vi "io.command-builder.DO.vi"(8 "error in":errorcluster, 9 "parsed dout state":cluster{"state":bool, "timeoutSeconds":u16}, 10 "IoConf in":T1={"ADDR"=0, "Label"="", "Type"=enum."DI", "Mode"=enum."RIO", "Value"="", "Tags"="", "calibration"=[]} {"calibration"."Y" format="%#.3f"; "calibration"."X" format="%#.3f"; "ADDR" format="%04d"}) -> (0 "error out":errorcluster, 2 "Frameless Command":string)   [LabVIEW 2024]
uses:
  controls/IONode.ctl
  controls/type.address.ctl
  controls/enum.io.type.ctl
  controls/enum.io.mode.ctl
  controls/typeXyPoint.ctl
  controls/enum.io-rio.ctl
  variantCtrlNumber.vi
panel:
  in  "Value in":cluster{"value":u8, "timeoutSeconds":u16}
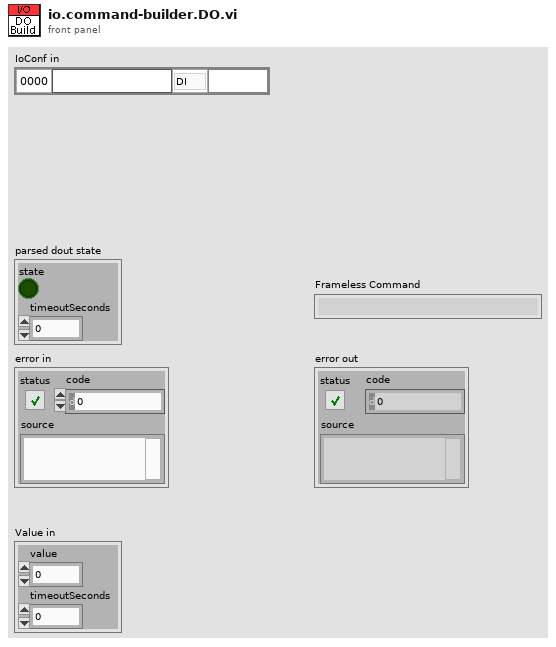
[diagram p1: front panel]
types:
  T1 = typedef "IONode.ctl" = cluster{"ADDR":T2, "Label":string, "Type":T3, "Mode":T4, "Value":string, "Tags":string, "calibration":T5[]}
  T2 = typedef "type.address.ctl" = u16
  T3 = typedef "enum.io.type.ctl" = enum16{"Type", "DI", "DO", "AI", "AO", "VL", "BUF"}
  T4 = typedef "enum.io.mode.ctl" = enum16{"Mode", "RIO", "SIM"}
  T5 = typedef "typeXyPoint.ctl" = cluster{"X":dbl, "Y":dbl}
  T6 = cluster{"DataSize":u8, "Address":u8, "Command(SET-DOUT)":u8, "Channel":u8, "DigVal":bool, "Timeout":u16}
  T7 = typedef "enum.io-rio.ctl" = enum16{"RIO_CALIBRATION"}
  T8 = cluster{"WRITE_DO":u8, "Address":T2, "Channel":u8, "value":u8, "timeoutSeconds":u16}
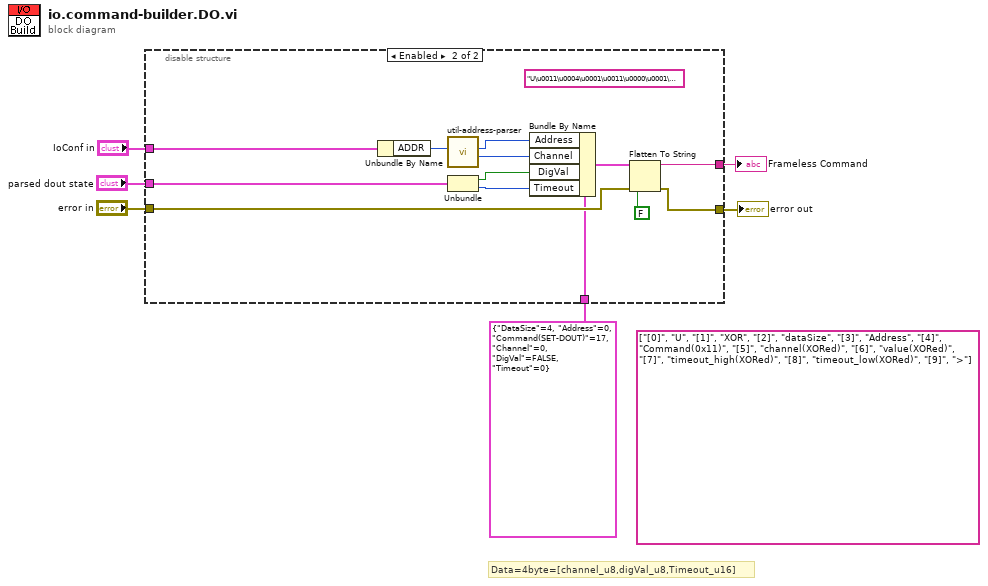
[diagram p0: block diagram]
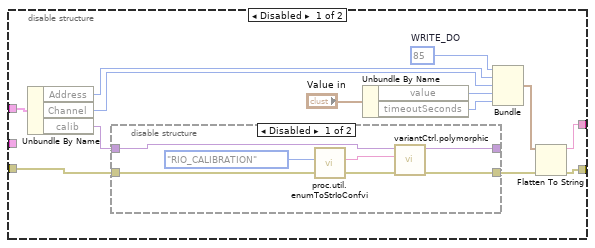
[diagram p2: hidden frame]
diagram:
  (unwired) string[][] [["[0]", "U"], ["[1]", "XOR"], ["[2]", "dataSize"], ["[3]", "Address"], ["[4]", "Command(0x11)"], ["[5]", "channel(XORed)"], ["[6]", "value(XORed)"], ["[7]", "timeout_high(XORed)"], ["[8]", "timeout_low(XORed)"], ["[9]", ">"]] ("Command To RIO")
  # "Data=4byte=[channel_u8,digVal_u8,Timeout_u16]"
  n1 = disable-structure shown="Enabled" {
    disable-tunnel: [w19 w40] -> w6
    disable-tunnel: "IoConf in" -> [w14 w39]
    disable-tunnel: "error in" -> [w12 w38]
    disable-tunnel: [w7 w37] -> w3
    disable-tunnel: "parsed dout state" -> [_ w31]
    disable-tunnel: T6 {"DataSize"=4, "Address"=0, "Command(SET-DOUT)"=17, "Channel"=0, "DigVal"=FALSE, "Timeout"=0} ("cluster") -> [_ w36]
    frame Disabled {
      w11 = u8 85  # WRITE_DO
      n2 = Unbundle By Name(w14) -> ("Address"=w17:T2, "Channel"=w18:u8, "calib"=w16:variant)
      n3 = disable-structure shown="Disabled" {
        disable-tunnel: w16 -> [w25 w27]
        disable-tunnel: [w24 w27] -> _
        disable-tunnel: [w23 w26] -> w15
        disable-tunnel: w12 -> [w20 w26]
        frame Disabled {
          n4 = call "proc.util.enumToStrIoConfvi.vi"("Step var"=enum.io-rio."RIO_CALIBRATION") -> ("String"=w22:string)  [unwired: 10 in]
          n5 = call-poly "variantCtrl.polymorphic.vi"("error in"=w20, "name in"=w22, "variant in"=w25) -> ("error out"=w23:errorcluster, "variant out"=w24:variant)  [unwired: 5 in, 2 out]
        }
        frame Enabled {
        }
      }
      n6 = Unbundle By Name("Value in") -> ("value"=w10:u8, "timeoutSeconds"=w9:u16)
      n7 = Bundle("WRITE_DO"=w11, "Address"=w17, "Channel"=w18, "value"=w10, "timeoutSeconds"=w9) -> (w8:T8)  [unwired: 1 in]
      n8 = Flatten To String(anything=w8, error in (no error)=w15) -> (data string=w19:string, error out=w7:errorcluster)  [unwired: 2 in, 1 out]
    }
    frame Enabled {
      (unwired) "U\u0011\u0004\u0001\u0011\u0000\u0001\u0000\u0000>" ("Command To RIO")
      n9 = Unbundle By Name(w39) -> ("ADDR"=w30:T2)
      n10 = call "util-address-parser.vi"("ADDR 2"=w30) -> ("Channel"=w29:u8, "Address"=w28:u8)  [unwired: 9 in]
      n11 = Unbundle(w31) -> ("state"=w34:bool, "timeoutSeconds"=w35:u16)
      n12 = Bundle By Name(cluster=w36, "Address"=w28, "Channel"=w29, "DigVal"=w34, "Timeout"=w35) -> (w33:T6)
      n13 = Flatten To String(anything=w33, prepend array or string size? (T)=FALSE, error in (no error)=w38) -> (data string=w40:string, error out=w37:errorcluster)  [unwired: 1 in, 1 out]
    }
  }
  "Frameless Command" <- w6
  "error out" <- w3
